vi "Multiple Write One Read(SubVI).vi"(0 "Channel in":u16, 5 "Messages to write":T1(array[cluster]), 7 "Mess 1 Passed":bool, 9 "ID":u32, 11 "error in":errorcluster, 12 "MaxRead":i32) -> (4 "Channel out":u16, 6 "Last Message":T2, 8 "Messages passed":bool, 15 "error out":errorcluster)   [LabVIEW 2023]
uses:
  072a70e8-6633-4579-be74-f239450be811.vi
  c67cbaf0-dbcc-43dd-b8b5-a9cde074df32.vi
  Communication/PCAN2023/PCAN API.lvlib
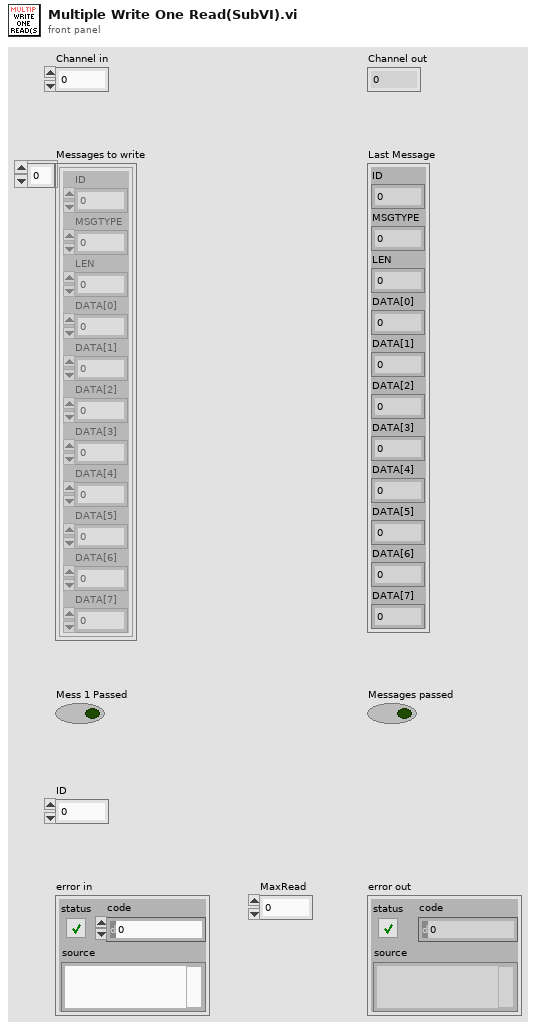
[diagram p1: front panel]
types:
  T1 = cluster{"ID":u32, "MSGTYPE":u8, "LEN":u8, "DATA[0]":u8, "DATA[1]":u8, "DATA[2]":u8, "DATA[3]":u8, "DATA[4]":u8, "DATA[5]":u8, "DATA[6]":u8, "DATA[7]":u8}[]
  T2 = cluster{"ID":u32, "MSGTYPE":u8, "LEN":u8, "DATA[0]":u8, "DATA[1]":u8, "DATA[2]":u8, "DATA[3]":u8, "DATA[4]":u8, "DATA[5]":u8, "DATA[6]":u8, "DATA[7]":u8}
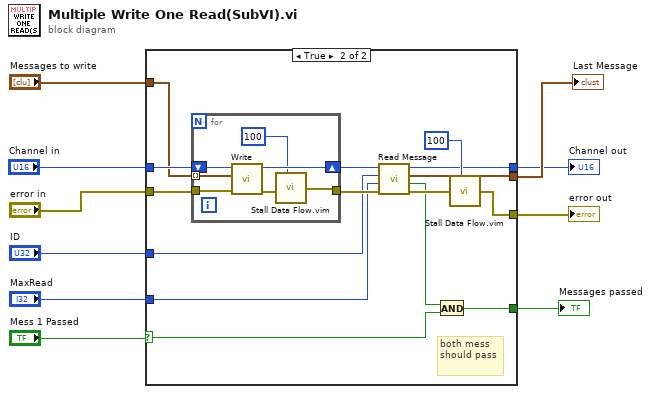
[diagram p0: block diagram]
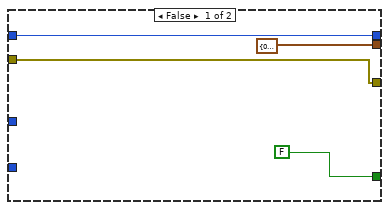
[diagram p2: hidden frame]
diagram:
  n1 = case shown="True" "Mess 1 Passed" {
    selector: "Mess 1 Passed" -> [_ w15]
    tunnel: "Channel in" -> [w13 w29]
    tunnel: "error in" -> [w11 w28]
    tunnel: [w11 w27] -> w2
    tunnel: [FALSE w24] -> w3
    tunnel: [w13 w21] -> w4
    tunnel: "Messages to write" -> [_ w26]
    tunnel: [T2 {"ID"=0, "MSGTYPE"=0, "LEN"=0, "DATA[0]"=0, "DATA[1]"=0, "DATA[2]"=0, "DATA[3]"=0, "DATA[4]"=0, "DATA[5]"=0, "DATA[6]"=0, "DATA[7]"=0} w16] -> w6
    tunnel: "ID" -> [_ w19]
    tunnel: "MaxRead" -> [_ w18]
    frame False {
    }
    frame True {
      # "both mess\nshould pass"
      n2 = for {
        tunnel: w26 -> [w32] mode=indexing
        shift-right: [w34] -> w23
        shift-left: w29 -> [w36]
        tunnel: w28 -> [w35]
        tunnel: [w33] -> w22
        n3 = call "Write.vi"("error in"=w35, "MessageBuffer"=w32, "Channel"=w36) -> ("error out"=w30:errorcluster, "Channel out"=w34:u16)  [unwired: 5 in, 2 out]
        n4 = call "Stall Data Flow.vim"("value in"=w30, "milliseconds to wait"=u32 100) -> ("value out"=w33:errorcluster)  [unwired: 1 out]
      }
      n5 = call "Read Message.vi"("error in"=w22, "MaxRead"=w18, "ID"=w19, "Channel in"=w23) -> ("error out"=w20:errorcluster, "Passed"=w17:bool, "Last Message"=w16:T2, "Channel out"=w21:u16)  [unwired: 3 in, 1 out]
      n6 = And(x=w17, y=w15) -> (x .and. y?=w24:bool)
      n7 = call "Stall Data Flow.vim"("value in"=w20, "milliseconds to wait"=u32 100) -> ("value out"=w27:errorcluster)  [unwired: 1 out]
    }
  }
  "Last Message" <- w6
  "Channel out" <- w4
  "Messages passed" <- w3
  "error out" <- w2
